vi "GET_Path.vi"(8 "error in (no error)":errorcluster, 11 "Icon Framework.lvclass in":refnum<class "Icon Framework.lvclass">) -> (0 "error out":errorcluster, 2 "Path":path, 3 "Icon Framework.lvclass out":refnum<class "Icon Framework.lvclass">)   [LabVIEW 2021, in "Icon Framework.lvclass"]
doc: "Returns the path to the used Template Layer glyph."
uses:
  Icon Framework.lvclass
  Icon Framework.lvclass/Icon Framework.ctl
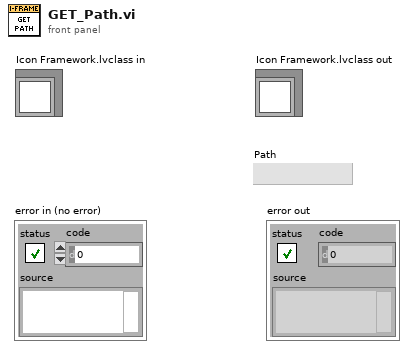
[diagram p1: front panel]
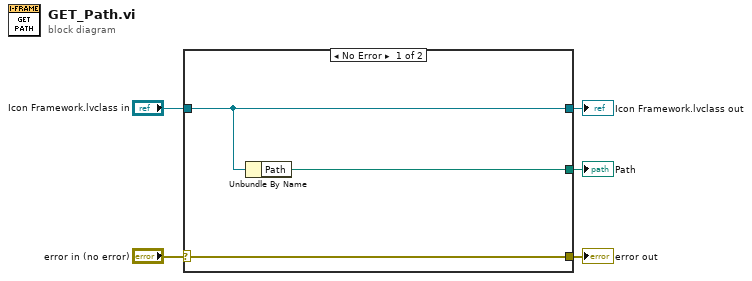
[diagram p0: block diagram]
diagram:
  n1 = case shown="No Error" "error in (no error)" {
    selector: "error in (no error)" -> [w8 w9]
    tunnel: [w8 w9] -> w4
    tunnel: [w7 w10] -> w2
    tunnel: "Icon Framework.lvclass in" -> [w7 w10]
    tunnel: [w6 _] -> w1
    frame No Error {
      n2 = Unbundle By Name(w7) -> ("Path"=w6:path)
    }
    frame Error {
    }
  }
  "error out" <- w4
  "Icon Framework.lvclass out" <- w2
  "Path" <- w1
